vi "Separate Array Values.vi"(0 "Input Array":dbl[](array[numeric])=[6.0, 3.9, -5.8, 0.0, -2.6, -1.0, 2.2, -4.3] format="%0.2f") -> (1 "Positive Array":dbl[](array[numeric]) format="%0.2f", 2 "Negative Array":dbl[](array[numeric]) format="%0.2f")   [LabVIEW 2014]
doc: "This VI takes an input array that contains a mixture of positive and negative values and separates that array into two smaller arrays - one containing just the negative values and one containing just the positive values. \n\nThe Initialize Array and Build Array functions are used and the For Loop sets its count by auto-indexing on the input array."
panel:
  # "This VI will sort the Input Array into two separate 1D arrays containing positive values and negative values."
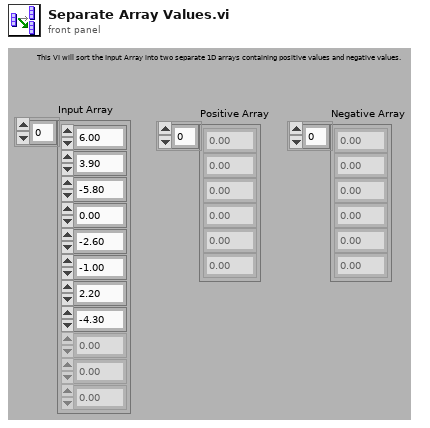
[diagram p1: front panel]
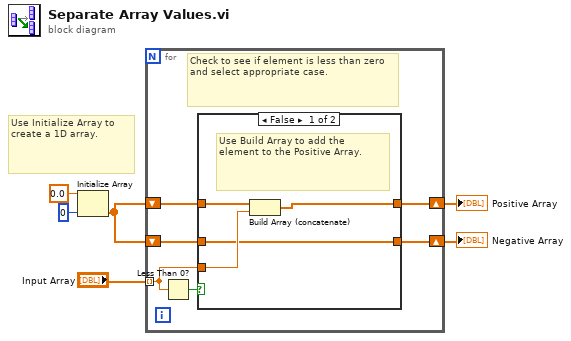
[diagram p0: block diagram]
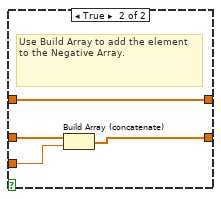
[diagram p2: hidden frame]
diagram:
  # "Use Initialize Array to create a 1D array."
  n1 = Initialize Array(0.0, 0) -> (w6:dbl[])
  n2 = for {
    shift-right: [w10] -> w2
    shift-left: w6 -> [w9]
    shift-right: [w7] -> w1
    shift-left: w6 -> [w8]
    tunnel: "Input Array" -> [w11] mode=indexing
    # "Check to see if element is less than zero and select appropriate case."
    n3 = Less Than 0?(x=w11) -> (x < 0?=w12:bool)
    n4 = case shown="False" w12 {
      tunnel: w11 -> [w14 w19]
      tunnel: [w15 w20] -> w10
      tunnel: w9 -> [w16 w20]
      tunnel: w8 -> [w13 w18]
      tunnel: [w13 w17] -> w7
      frame False {
        # "Use Build Array to add the element to the Positive Array."
        n5 = Build Array (concatenate)(w16, w14) -> (w15:dbl[])
      }
      frame True {
        # "Use Build Array to add the element to the Negative Array."
        n6 = Build Array (concatenate)(w18, w19) -> (w17:dbl[])
      }
    }
  }
  "Positive Array" <- w2
  "Negative Array" <- w1
